vi "总氮单步调试对话框.vi"() -> ()   [LabVIEW 2016, in "斯坦道总氮.lvlib"]
panel:
  in  "退出":bool
  in  "启动":bool
  in  "总磷氨氮调试":u16[](xcontrol)
  # "总氮单步调试界面"
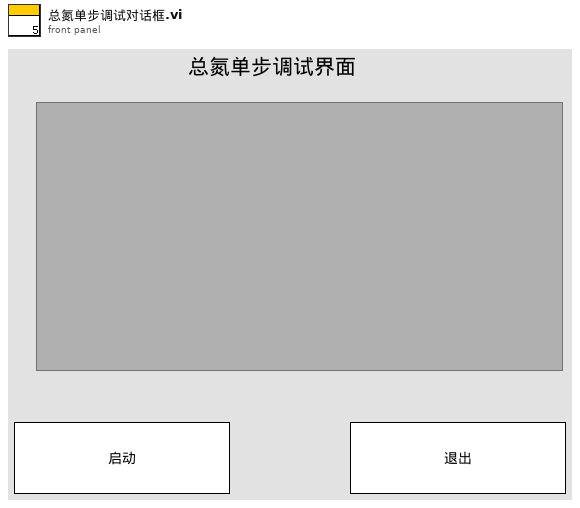
[diagram p1: front panel]
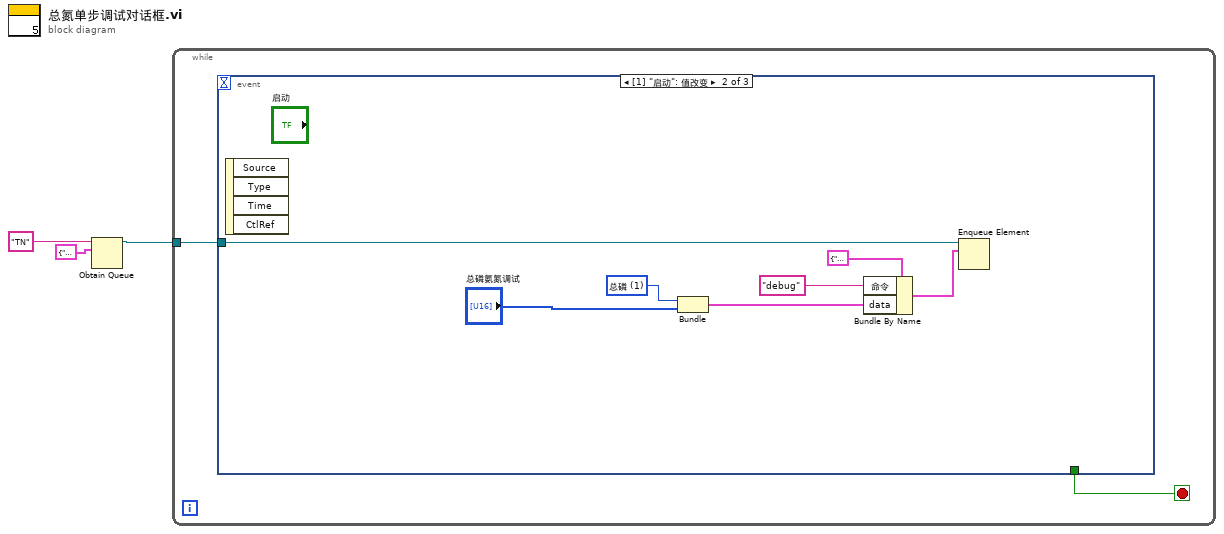
[diagram p0: block diagram]
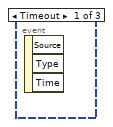
[diagram p2: hidden frame]
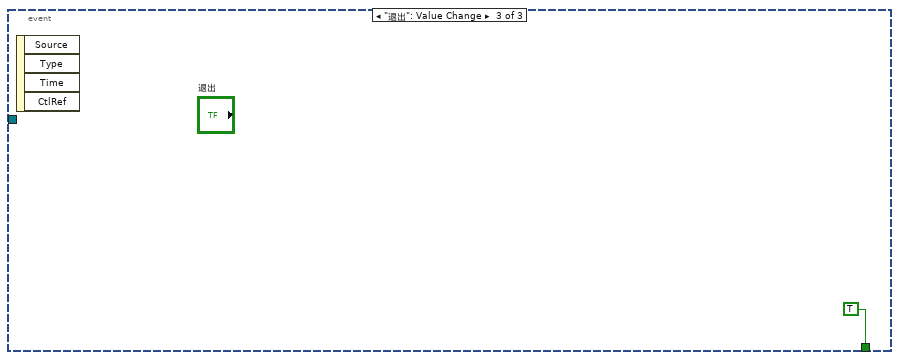
[diagram p3: hidden frame]
diagram:
  n1 = Obtain Queue(name (unnamed)="TN" ("名称（未命名）"), element data type=cluster{"命令":string, "data":variant} {"命令"="", "data"=variant}) -> (queue out=w1:refnum<queue>)  [unwired: 3 in, 2 out]
  n2 = while {
    tunnel: w1 -> [w5]
    stop <- w4 stop-if-true
    n3 = event shown="[1] \"启动\": 值改变" {
      selector: _ -> [_ _ _]
      dyn-events: _ -> [_ _ _]
      timeout: _ -> [_ _ _]
      tunnel: w5 -> [_ w7 _]
      tunnel: [_ _ TRUE] -> w4
      event Timeout {
        n4 = event-data() -> ()  [unwired: 1 in, 3 out]
      }
      event "启动": Value Change {
        w9 = u16 1 items=["总磷"=1, "氨氮"=3] ("站号")
        n5 = event-data() -> ()  [unwired: 1 in, 4 out]
        n6 = Bundle("站号"=w9, "总磷氨氮调试"="总磷氨氮调试") -> (w8:cluster{"站号":u16, "总磷氨氮调试":u16[]})  [unwired: 1 in]
        n7 = Bundle By Name(cluster=cluster{"命令":string, "data":variant} {"命令"="", "data"=variant} ("元素"), "命令"="debug", "data"=w8) -> (w10:cluster{"命令":string, "data":variant})
        n8 = Enqueue Element(queue=w7, element=w10) -> ()  [unwired: 2 in, 3 out]
      }
      event "退出": Value Change {
        n9 = event-data() -> ()  [unwired: 1 in, 4 out]
      }
    }
  }
